vi "查询上序合格03.vi"(8 "error in (no error)":errorcluster, 11 "产品ID":string) -> (0 "error out":errorcluster, 2 "合格02":bool)   [LabVIEW 2011]
uses:
  <vilib>/Utility/error.llb/whitespace.ctl
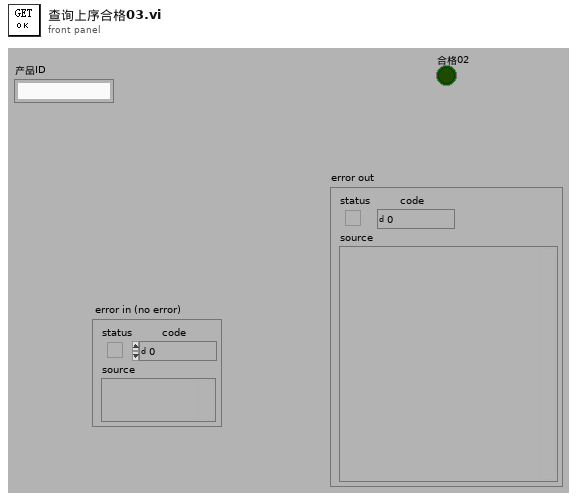
[diagram p1: front panel]
types:
  T1 = typedef "whitespace.ctl" = u16
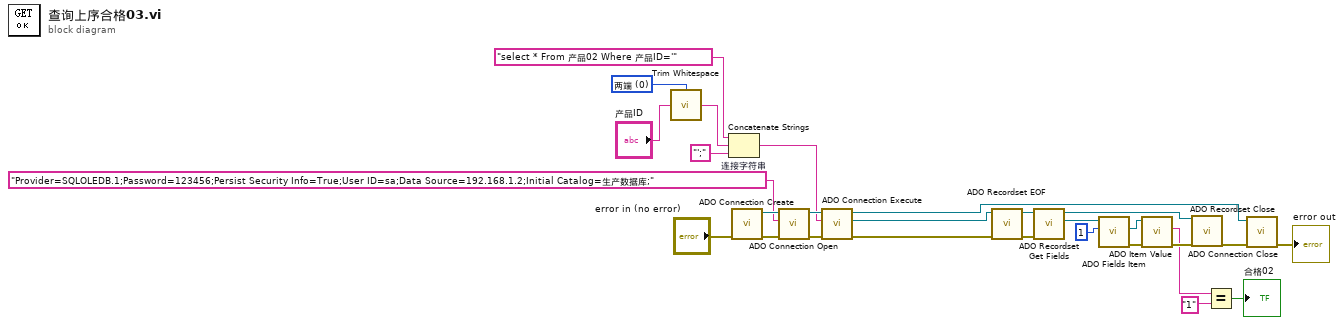
[diagram p0: block diagram]
diagram:
  w15 = T1 0 items=["两端", "字符串首端", "字符串末端"] ("location (both)")
  n1 = call <vilib>:"Trim Whitespace.vi"("string"="产品ID", "location (both)"=w15) -> ("trimmed string"=w16:string)
  n2 = Concatenate Strings "连接字符串"("select * From 产品02 Where 产品ID='" ("字符串 2"), w16, "';" ("字符串 2")) -> (w14:string)
  n3 = call "ADO Connection Create.vi"("error in (no error)"="error in (no error)") -> ("error out"=w27:errorcluster, "ADODB._Connection Out"=w28:refnum<k7>)  [unwired: 9 out]
  n4 = call "ADO Connection Open.vi"("error in (no error)"=w27, "ConnectionString"="Provider=SQLOLEDB.1;Password=123456;Persist Security Info=True;User ID=sa;Data Source=192.168.1.2;Initial Catalog=生产数据库;" ("字符串 2"), "ADODB._Connection In"=w28) -> ("error out"=w26:errorcluster, "ADODB._Connection Out"=w25:refnum<k7>)  [unwired: 7 out]
  n5 = call "ADO Connection Execute.vi"("error in (no error)"=w26, "CommandText"=w14, "ADODB._Connection In"=w25) -> ("error out"=w22:errorcluster, "RecordSet"=w23:refnum<k7>, "ADODB._Connection Out"=w20:refnum<k7>)  [unwired: 6 out]
  n6 = call "ADO Recordset EOF.vi"("error in (no error)"=w22, "ADODB._Recordset In"=w23) -> ("error out"=w10:errorcluster, "ADODB._Recordset Out"=w11:refnum<k7>)  [unwired: 8 out]
  n7 = call "ADO Recordset Get Fields.vi"("error in (no error)"=w10, "ADODB._Recordset In"=w11) -> ("Fields Out"=w7:refnum<k7>, "ADODB._Recordset Out"=w9:refnum<k7>)  [unwired: 8 out]
  n8 = call "ADO Fields Item.vi"("Index"=1, "Fields In"=w7) -> ("error out"=w5:errorcluster, "Item Out"=w4:refnum<k7>)  [unwired: 1 in, 7 out]
  n9 = call "ADO Item Value.vi"("error in (no error)"=w5, "Item In"=w4) -> ("error out"=w8:errorcluster, "Value"=w3:string)  [unwired: 8 out]
  n10 = call "ADO Recordset Close.vi"("ADODB._Recordset In"=w9, "error in (no error)"=w8) -> ("error out"=w21:errorcluster)  [unwired: 17 out]
  n11 = Equal?(x=w3, y="1") -> (x = y?=→"合格02":bool)
  n12 = call "ADO Connection Close.vi"("error in (no error)"=w21, "ADODB._Connection In"=w20) -> ("error out"=→"error out":errorcluster)  [unwired: 9 out]
